vi "BC Major Frame Start.vi"(8 "error in (no error)":errorcluster, 11 "Bus Controller in":refnum<class "Bus Controller.lvclass">) -> (0 "error out":errorcluster, 3 "Bus Controller out":refnum<class "Bus Controller.lvclass">)   [LabVIEW 2020, in "Unit Tests.lvlib" / "Bus Controller.lvclass"]
uses:
  Bus Controller.lvclass
  Bus Controller.lvclass/Bus Controller.ctl
  Frames & Messages/TypeDefs/BC Op Codes - Verbose.ctl
  Frames & Messages/TypeDefs/BC Condition Codes.ctl
  <vilib>/addons/_JKI Toolkits/Caraya/classes/Assert/Assert True.vi
  Dependencies/FPGA Interface/FPGA Interface.lvclass
  BCI-1553 API.lvlib
  <vilib>/addons/_JKI Toolkits/Caraya/classes/Assert/Assert.lvclass
  <vilib>/addons/_JKI Toolkits/Caraya/classes/Test/Test.lvclass
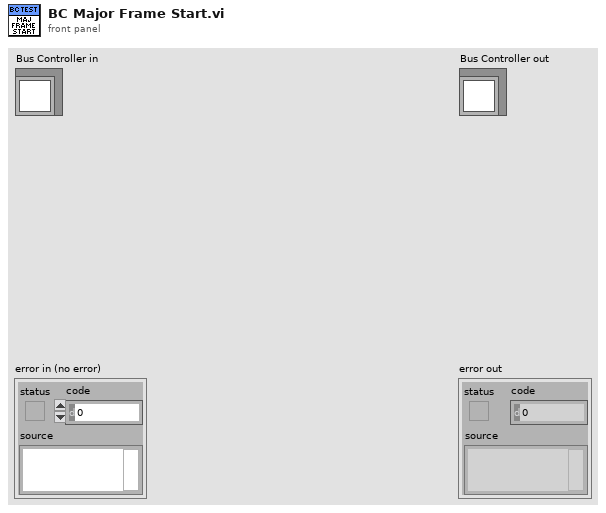
[diagram p1: front panel]
types:
  T1 = typedef "BCI-1553 API.lvlib/BC Op Codes - Verbose.ctl" = enum16{"EXECUTE MSG", "EXECUTE MSG GO", "JUMP", "CALL SUBROUTINE", "RETURN", "INTERRUPT REQUEST", "HALT", "DELAY", "WAIT FRAME TIMER = 0", "COMPARE FRAME TIMER", "COMPARE MSG TIMER", "LOAD TIME TAG CTR", "LOAD TIME TAG CTR HI", "LOAD FRAME TIMER", "START FRAME TIMER", "PUSH TIME TAG COUNT", "PUSH TIME TAG COUNT HI", "PUSH TIME TAG COUNT BOTH", "PUSH BLOCK STATUS WORD", "PUSH CURRENT VALUE", "PUSH INDIRECT", "WAIT EXT TRIGGER", "EXECUTE AND FLIP", "EXECUTE, FLIP, GO", "WRITE VALUE TO WMI", "WRITE VALUE TO MEM", "DECREMENT RAM, SKIP", "FLAG"}
  T2 = typedef "BCI-1553 API.lvlib/BC Condition Codes.ctl" = enum16{"GP0 == 1 || LT", "GP1 == 1 || NE", "GP2 == 1", "GP3 == 1", "GP4 == 1", "GP5 == 1", "GP6 == 1", "GP7 == 1", "NORESP", "FMTERR", "GOODBLOCK", "MSKSTATSET", "BADMSG", "1RETRY", "2RETRY", "ALWAYS"}
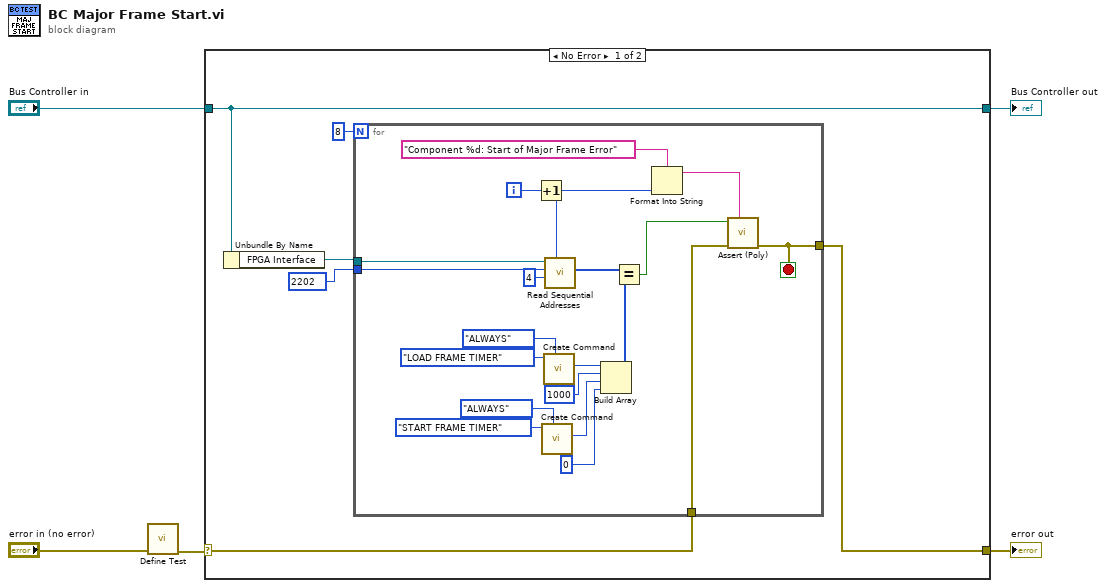
[diagram p0: block diagram]
diagram:
  n1 = call <vilib>:"Define Test.vi"("error in (no error)"="error in (no error)") -> ("error out"=w2:errorcluster)  [unwired: 9 in, 1 out]
  n2 = case shown="No Error" w2 {
    selector: w2 -> [w8 w33]
    tunnel: [w7 w33] -> w5
    tunnel: [w11 w32] -> w3
    tunnel: "Bus Controller in" -> [w11 w32]
    frame No Error {
      n3 = Unbundle By Name(w11) -> ("FPGA Interface"=w10:refnum<class "FPGA Interface.lvclass">)
      n4 = for {
        N: 8 -> [_]
        tunnel: w10 -> [w31]
        tunnel: u16 2202 -> [w28]
        tunnel: [w13] -> w7
        tunnel: w8 -> [w12]
        i -> [w29]
        stop <- w13 stop-if-true
        n5 = Increment(x=w29) -> (x+1=w26:i32)
        n6 = call "Create Command.vi"("Condition"=BC_Condition_Codes."ALWAYS", "Op Code"=BC_Op_Codes_-_Verbose."START FRAME TIMER") -> ("Instruction"=w19:u16)  [unwired: 8 in, 1 out]
        n7 = call "Create Command.vi"("Condition"=BC_Condition_Codes."ALWAYS", "Op Code"=BC_Op_Codes_-_Verbose."LOAD FRAME TIMER") -> ("Instruction"=w21:u16)  [unwired: 8 in, 1 out]
        n8 = call-dynamic "Read Sequential Addresses.vi"("Target IC (1-8)"=w26, "Addresses to Read"=u16 4, "Starting Address"=w28, "FPGA Interface in"=w31) -> ("Data"=w16:u16[])  [unwired: 6 in, 1 out]
        n9 = Build Array(w21, u16 1000 ("x"), w19, u16 0 ("x")) -> (w17:u16[])
        n10 = Equal?(x=w16, y=w17) -> (x = y?=w15:bool)
        n11 = Format Into String(format string="Component %d: Start of Major Frame Error" ("custom report message (\"\")"), w26) -> (resulting string=w14:string)  [unwired: 2 in, 1 out]
        n12 = call-poly <vilib>:"Assert (Poly).vi"("Label"=w14, "error in (no error)"=w12, "True?"=w15) -> ("error out"=w13:errorcluster)  [unwired: 7 in, 1 out]
      }
    }
    frame Error {
    }
  }
  "error out" <- w5
  "Bus Controller out" <- w3
